vi "XMLGetItemInfo.vi"(8 "error in (no error)":errorcluster, 11 "ArrayOfNodes":refnum<k20>[](array[refnum])) -> (0 "error out":errorcluster, 3 "Array":cluster{"Name":string, "Value":string}[](array[cluster]))   [LabVIEW 2014, in "OPCUA XML(dev).lvlib"]
uses:
  OPCUA XML(dev).lvlib
  <resource>/objmgr/DOMUserDefRef.rc
  <vilib>/xml/NI_XML.lvlib
  <vilib>/xml/Close Reference(Node).vi
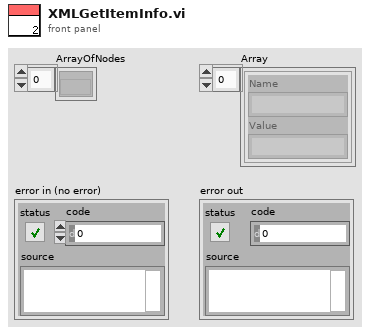
[diagram p1: front panel]
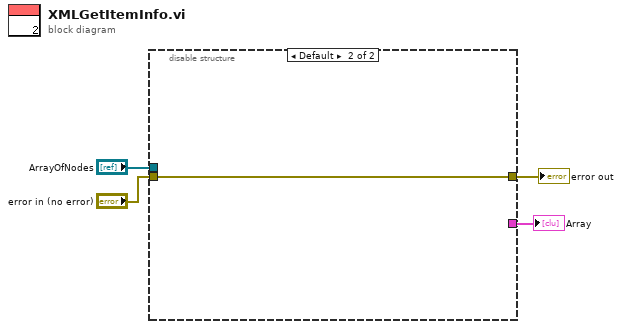
[diagram p0: block diagram]
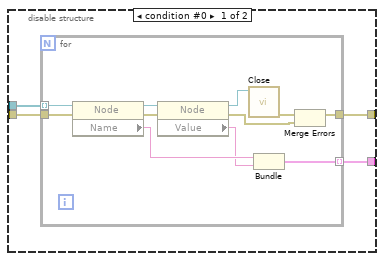
[diagram p2: hidden frame]
diagram:
  n1 = disable-structure shown="Default" {
    disable-tunnel: [w8 _] -> w4
    disable-tunnel: [w7 w20] -> w3
    disable-tunnel: "error in (no error)" -> [w6 w20]
    disable-tunnel: "ArrayOfNodes" -> [w5 _]
    frame condition #0 {
      n2 = for {
        tunnel: [w10] -> w7
        tunnel: [w13] -> w8 mode=indexing
        tunnel: w5 -> [w12] mode=indexing
        tunnel: w6 -> [w11]
        n3 = property class="Node"(reference=w12, error in=w11) -> (reference out=w16:refnum<k20>, error out=w18:errorcluster, "Name"=w15:string)
        n4 = property class="Node"(reference=w16, error in=w18) -> (reference out=w17:refnum<k20>, error out=w9:errorcluster, "Value"=w14:string)
        n5 = call-poly <vilib>:"Close.vi"("node"=w17) -> ("error out"=w19:errorcluster)  [unwired: 1 in, 7 out]
        n6 = Bundle("Name"=w15, "Value"=w14) -> (w13:cluster{"Name":string, "Value":string})  [unwired: 1 in]
        n7 = Merge Errors(w19, w9) -> (w10:errorcluster)
      }
    }
    frame condition #1 (active) {
    }
  }
  "Array" <- w4
  "error out" <- w3
